vi "init.vi"(8 "error in (no error)":errorcluster, 9 "Number of Iterations":T1, 10 "Inputs to Guassian Noise Wave":T2, 11 "GuassianNoiseWave in":refnum<class "GuassianNoiseWave.lvclass">) -> (0 "error out":errorcluster, 3 "GuassianNoiseWave out":refnum<class "GuassianNoiseWave.lvclass">)   [LabVIEW 2015, in "GuassianNoiseWave.lvclass"]
uses:
  GuassianNoiseWave.lvclass
  Typedefs/GuassianNoiseWaveInput.ctl
  Typedefs/Iterations.ctl
  GuassianNoiseWave.lvclass/GuassianNoiseWave.ctl
  Typedefs/FAMTTypedefs.lvlib
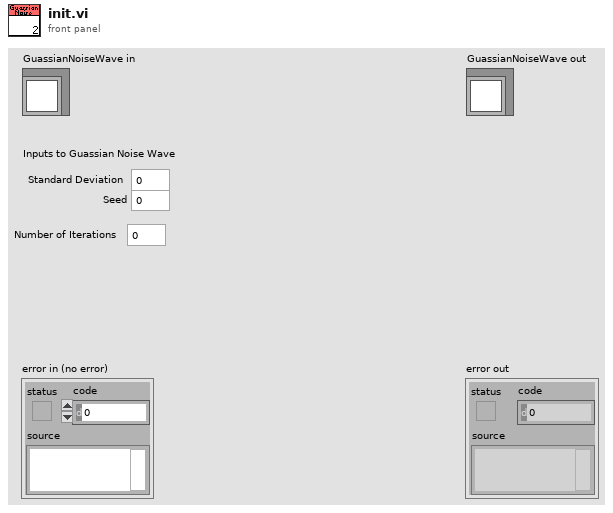
[diagram p1: front panel]
types:
  T1 = typedef "FAMTTypedefs.lvlib/Iterations.ctl" = i32
  T2 = typedef "FAMTTypedefs.lvlib/GuassianNoiseWaveInput.ctl" = cluster{"Seed":i32, "Standard Deviation":dbl}
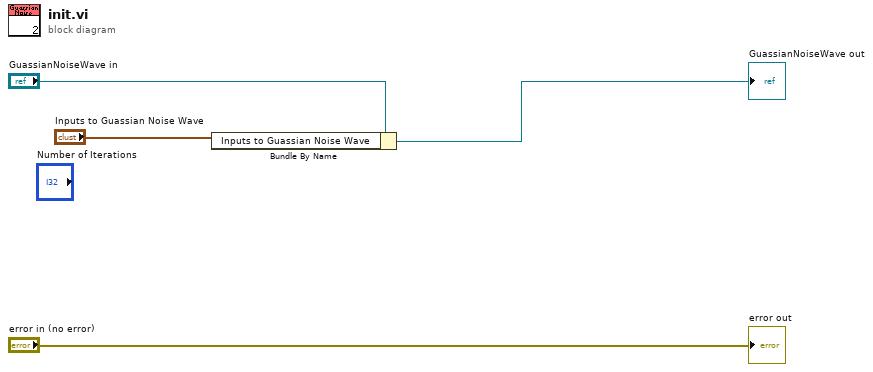
[diagram p0: block diagram]
diagram:
  n1 = Bundle By Name(cluster="GuassianNoiseWave in", "Inputs to Guassian Noise Wave"="Inputs to Guassian Noise Wave") -> (→"GuassianNoiseWave out":refnum<class "GuassianNoiseWave.lvclass">)
  "error out" <- "error in (no error)"
